vi "Take Snapshot.vi"(8 "error in (no error)":errorcluster, 9 "Timeout (ms)":i32, 11 "Camera in":refnum<class "Camera.lvclass">) -> (0 "error out":errorcluster, 2 "New Buffer":refnum<class "Buffer.lvclass">, 3 "Camera":refnum<class "Camera.lvclass">)   [LabVIEW 2020, in "Camera.lvclass"]
uses:
  Camera.lvclass
  Buffer/Buffer.lvclass
  Camera.lvclass/Camera.ctl
  Buffer/Buffer.lvclass/Buffer.ctl
  bin/gindustrialcam_32-1.dll
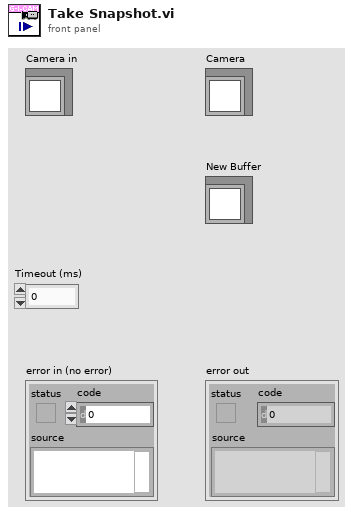
[diagram p1: front panel]
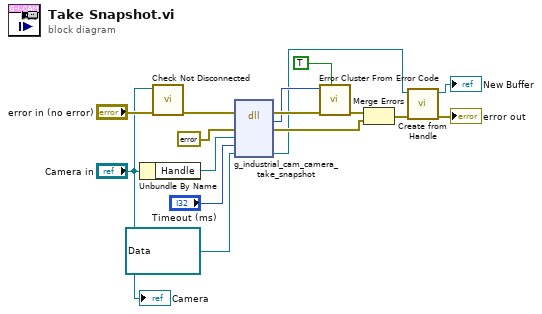
[diagram p0: block diagram]
diagram:
  n1 = Unbundle By Name("Camera in") -> ("Handle"=w9:refnum<data-value>)
  n2 = call "Check Not Disconnected.vi"("error in (no error)"="error in (no error)", "Camera in"="Camera in") -> ("error out"=w2:errorcluster)  [unwired: 9 in]
  n3 = dll-call lib="C:/Workspace/SSDC/g-industrial-camera/LabVIEW/g_industrial_cam/bin/gindustrialcam_*-1.*" fn="g_industrial_cam_camera_take_snapshot"(error in=w2, "err"=errorcluster {"status"=FALSE, "code"=0, "source"=""} ("error constant"), "cam_edvr"=w9, "timeout"="Timeout (ms)", "buffer_edvr"=refnum<data-value> refnum ("Handle")) -> (error out=w15:errorcluster, "Mg_Error"=w14:i32, "err"=w12:errorcluster, "buffer_edvr"=w6:refnum<data-value>)  [unwired: 4 in, 1 out]
  n4 = call <vilib>:"Error Cluster From Error Code.vi"("show call chain? (False)"=TRUE, "error in (no error)"=w15, "error code (0)"=w14) -> ("error out"=w13:errorcluster)  [unwired: 6 in]
  n5 = Merge Errors(w13, w12) -> (w5:errorcluster)
  n6 = call "Create from Handle.vi"("error in (no error)"=w5, "Handle"=w6) -> ("error out"=→"error out":errorcluster, "Buffer out"=→"New Buffer":refnum<class "Buffer.lvclass">)  [unwired: 8 in]
  "Camera" <- "Camera in"
